vi "Preset_Edit.vi"() -> ()   [LabVIEW 2020, in "Gviewer.lvclass"]
doc: "Andre Koelewijn, 20 jan 2021\n\nEdit TAGs to display"
uses:
  Gviewer.lvclass
  controls/EditTagOneTag.ctl
  controls/Typedef_Gserver-Replies.ctl
  controls/Typedef_ServerActions.ctl
  DBAL/controls/DBAL_TAGprops.ctl
  DBAL/controls/DBAL_TAGpropEdit.ctl
  Common/controls/typedef_com_TagProp.ctl
  <vilib>/Utility/miscctls.llb/LVPointTypeDef.ctl
panel:
  in  "Exit_event":bool
  out "tag-info":string
  in  "TAGproperties":T1 {"TAGprop"."TagFunc" format="%08x"; "TAGprop"."RangeL" format="%.2f"; "TAGprop"."RangeH" format="%.2f"}
  in  "GViewer-Queue":refnum<queue>
  in  "SaveAs":bool
  in  "Save":bool
  in  "Cancel":bool
  in  "Selector":i32[](listbox)
  in  "Presets":T4[](array[typedef]) {"max" format="%#_6p"; "min" format="%#_6p"}
  # "Tag name"
  # "scale L"
  # "scale H"
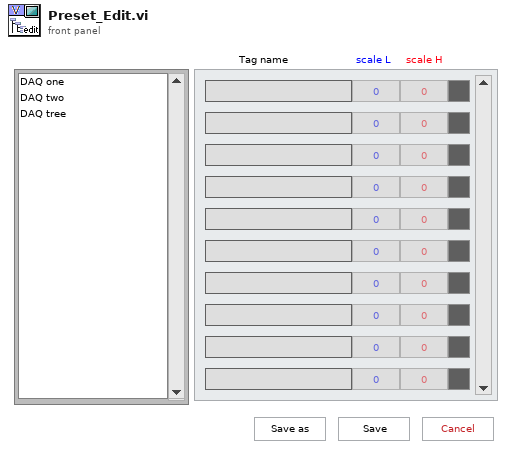
[diagram p1: front panel]
types:
  T1 = typedef "DBAL_TAGprops.ctl" = T2[]
  T2 = typedef "DBAL_TAGpropEdit.ctl" = cluster{"TAG":string, "Qtype":string, "TAGprop":T3}
  T3 = typedef "typedef_com_TagProp.ctl" = cluster{"Description":string, "EngUnits":string, "RangeH":dbl, "RangeL":dbl, "Resolution":i32, "Obsolete":bool, "ChangeDate":timestamp, "ChangeSource":string, "ChangeReason":string, "TagFunc":u32}
  T4 = typedef "EditTagOneTag.ctl" = cluster{"TAG":string, "min":dbl, "max":dbl, "Color":u32}
  T5 = typedef "LVPointTypeDef.ctl" = cluster{"Horizontal":i16, "Vertical":i16}
  T6 = typedef "Typedef_ServerActions.ctl" = enum16{"GraphUpdate", "SendAllTags", "SendIniPath", "SetGeneralOptions", "EditTagsOpen", "EditTagsClose", "NewTagSelection", "ExitGraph"}
  T7 = typedef "Typedef_Gserver-Replies.ctl" = cluster{"ServerActions":T6, "data":variant, "Source":string, "Time Stamp":timestamp}
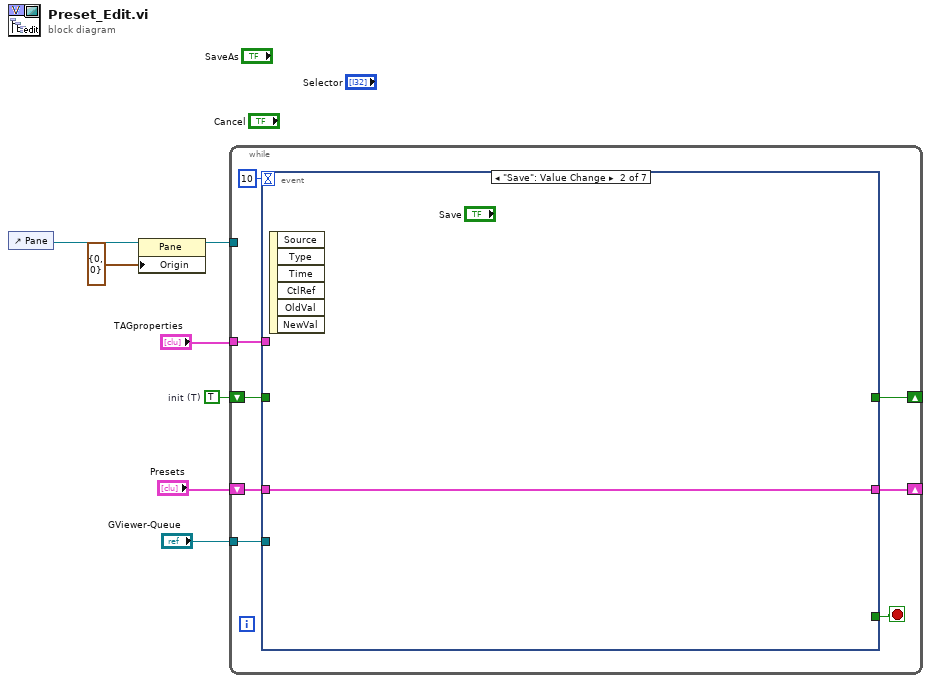
[diagram p0: block diagram]
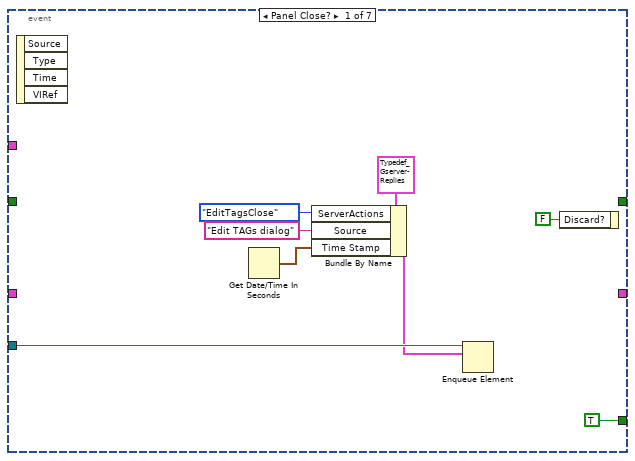
[diagram p2: hidden frame]
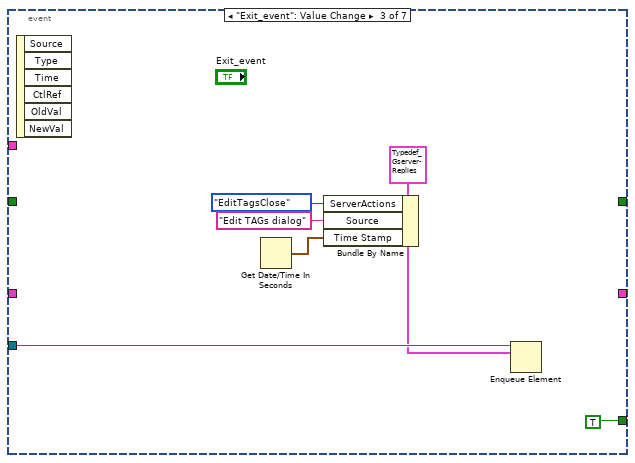
[diagram p3: hidden frame]
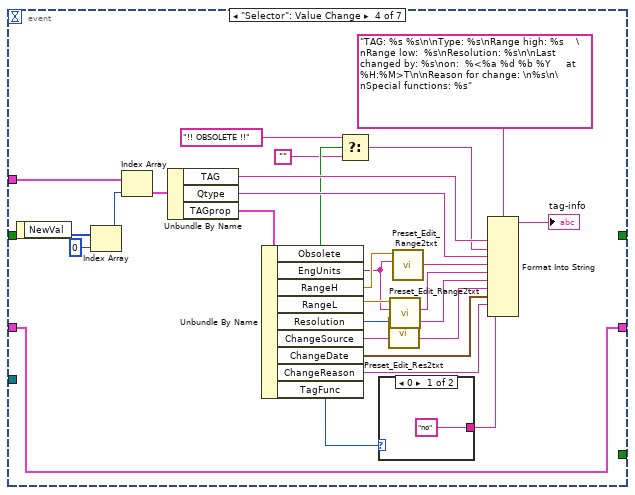
[diagram p4: hidden frame]
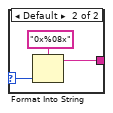
[diagram p5: hidden frame]
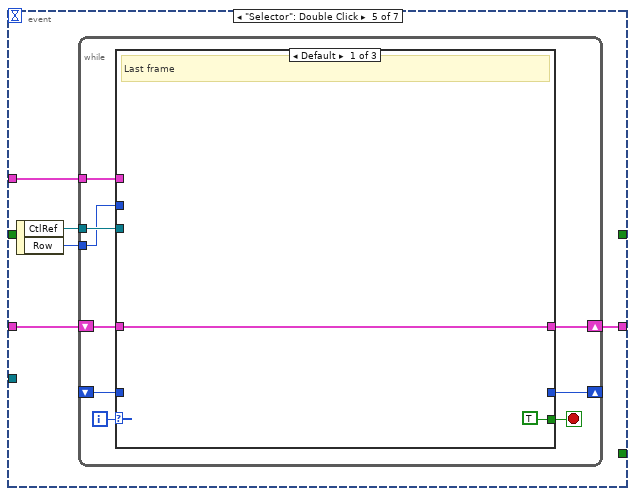
[diagram p6: hidden frame]
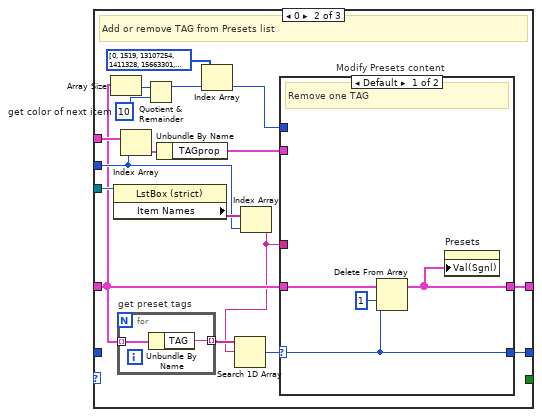
[diagram p7: hidden frame]
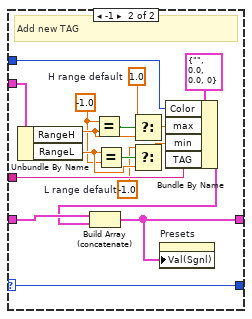
[diagram p8: hidden frame]
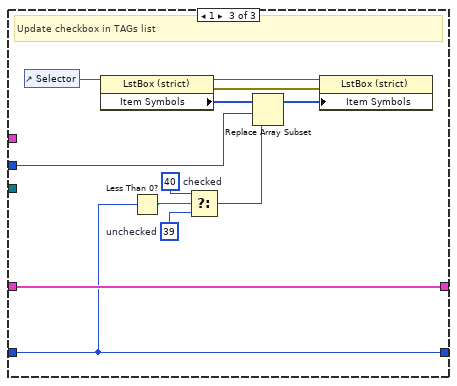
[diagram p9: hidden frame]
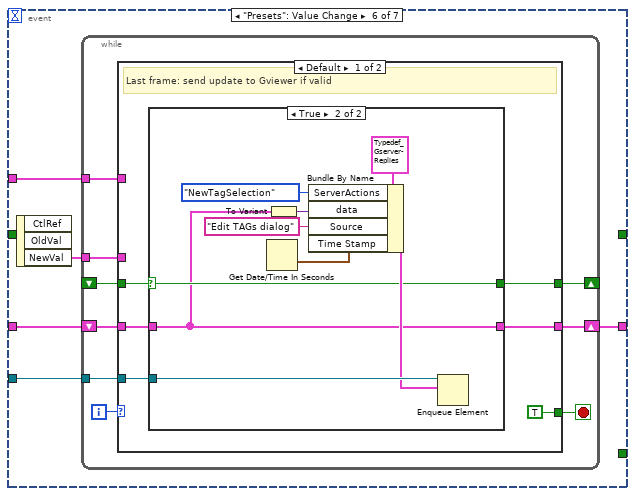
[diagram p10: hidden frame]
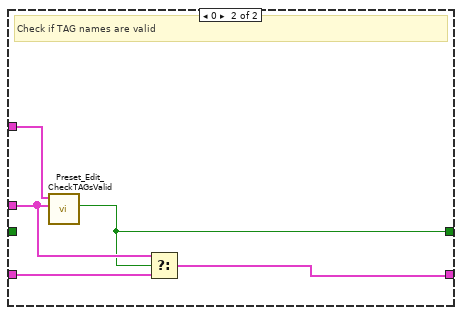
[diagram p12: hidden frame]
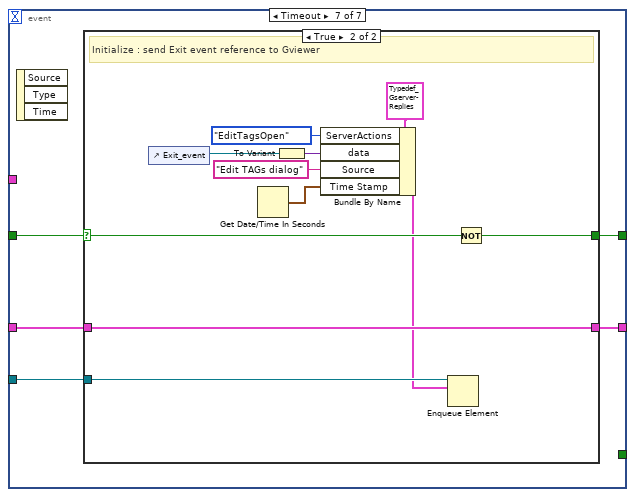
[diagram p13: hidden frame]
diagram:
  w1 = TRUE  # init (T)
  n1 = control-ref of="Pane"() -> (w6:refnum<vi>)
  n2 = property class="Pane"(reference=w6, "Origin"=T5 {"Horizontal"=0, "Vertical"=0}) -> (reference out=w5:refnum<vi>)  [unwired: 1 in, 1 out]
  n3 = while {
    tunnel: w5 -> [_]
    tunnel: "TAGproperties" -> [w13]
    tunnel: "GViewer-Queue" -> [w10]
    shift-right: [w11] -> _
    shift-left: "Presets" -> [w12]
    shift-right: [w8] -> _
    shift-left: w1 -> [w9]
    stop <- w15 stop-if-true
    n4 = event shown="[1] \"Save\": Value Change" {
      selector: _ -> [_ _ _ _ _ _ _]
      dyn-events: _ -> [_ _ _ _ _ _ _]
      timeout: 10 -> [_ _ _ _ _ _ _]
      tunnel: [TRUE _ TRUE _ _ _ _] -> w15
      tunnel: w13 -> [_ _ _ w57 w62 w130 _]
      tunnel: w12 -> [_ w24 _ w31 w64 w134 w169]
      tunnel: [_ w24 _ w31 w63 w133 w168] -> w11
      tunnel: w10 -> [w17 _ w29 _ _ w132 w166]
      tunnel: w9 -> [_ _ _ _ _ _ w170]
      tunnel: [_ _ _ _ _ _ w167] -> w8
      event Panel Close? {
        n5 = event-data() -> ()  [unwired: 1 in, 4 out]
        n6 = Get Date/Time In Seconds() -> (seconds since 1Jan1904=w21:timestamp)
        n7 = Bundle By Name(cluster=T7 {"ServerActions"=enum."GraphUpdate", "data"=variant, "Source"="", "Time Stamp"=timestamp(0 s since 1904-01-01)} ("element"), "ServerActions"=Typedef_ServerActions."EditTagsClose", "Source"="Edit TAGs dialog", "Time Stamp"=w21) -> (w16:T7)
        n8 = Enqueue Element(queue=w17, element=w16) -> ()  [unwired: 2 in, 3 out]
        n9 = event-data("Discard?"=FALSE) -> ()  [unwired: 1 in, 1 out]
      }
      event "Save": Value Change {
        n10 = event-data() -> ()  [unwired: 1 in, 6 out]
      }
      event "Exit_event": Value Change {
        w25 = T7 {"ServerActions"=enum."GraphUpdate", "data"=variant, "Source"="", "Time Stamp"=timestamp(0 s since 1904-01-01)} ("element")
        n11 = event-data() -> ()  [unwired: 1 in, 6 out]
        n12 = Get Date/Time In Seconds() -> (seconds since 1Jan1904=w26:timestamp)
        n13 = Bundle By Name(cluster=w25, "ServerActions"=Typedef_ServerActions."EditTagsClose", "Source"="Edit TAGs dialog", "Time Stamp"=w26) -> ()  [unwired: 1 out]
        n14 = Enqueue Element(queue=w29, element=w25) -> ()  [unwired: 2 in, 3 out]
      }
      event "Selector": Value Change {
        n15 = event-data() -> ("NewVal"=w56:i32[])  [unwired: 1 in]
        n16 = Index Array(array=w56, index=0) -> (element=w54:i32)
        n17 = Index Array(array=w57, index=w54) -> (element=w53:T2)
        n18 = Unbundle By Name(w53) -> ("TAG"=w44:string, "Qtype"=w50:string, "TAGprop"=w52:T3)
        n19 = Unbundle By Name(w52) -> ("Obsolete"=w43:bool, "EngUnits"=w37:string, "RangeH"=w39:dbl, "RangeL"=w38:dbl, "Resolution"=w35:i32, "ChangeSource"=w49:string, "ChangeDate"=w48:timestamp, "ChangeReason"=w47:string, "TagFunc"=w33:u32)
        n20 = Select(t="!! OBSOLETE !!" ("format string"), s=w43, f="") -> (s? t:f=w42:string)
        n21 = case shown="0" w33 {
          selector: w33 -> [_ w60]
          tunnel: ["no" w59] -> w32
          frame 0 {
          }
          frame Default {
            n22 = Format Into String(format string="0x%08x", w60) -> (resulting string=w59:string)  [unwired: 2 in, 1 out]
          }
        }
        n23 = call "Preset_Edit_Res2txt.vi"("Resolution"=w35) -> ("Resolution text"=w34:string)  [unwired: 10 in]
        n24 = call "Preset_Edit_Range2txt.vi"("Engineering units"=w37, "Range"=w38) -> ("RangeInfo"=w36:string)  [unwired: 9 in]
        n25 = call "Preset_Edit_Range2txt.vi"("Engineering units"=w37, "Range"=w39) -> ("RangeInfo"=w40:string)  [unwired: 9 in]
        n26 = Format Into String(format string="TAG: %s %s\n\nType: %s\nRange high: %s    \nRange low:  %s\nResolution: %s\n\nLast changed by: %s\non:  %<%a %d %b %Y     at  %H:%M>T\n\nReason for change: \n%s\n\nSpecial functions: %s", w44, w42, w50, w40, w36, w34, w49, w48, w47, w32) -> (resulting string=→"tag-info":string)  [unwired: 2 in, 1 out]
      }
      event "Selector": Double Click {
        n27 = event-data() -> ("CtlRef"=w66:refnum<vi>, "Row"=w65:i32)  [unwired: 1 in]
        n28 = while {
          tunnel: w66 -> [w71]
          tunnel: w65 -> [w70]
          shift-right: [w73] -> w63
          shift-left: w64 -> [w74]
          tunnel: w62 -> [w72]
          shift-right: [w69] -> _
          shift-left: _ -> [w68]
          i -> [w75]
          stop <- w67 stop-if-true
          n29 = case shown="Default" w75 {
            tunnel: w74 -> [w76 w83 w123]
            tunnel: [w76 w81 w123] -> w73
            tunnel: w72 -> [_ w87 _]
            tunnel: w71 -> [_ w88 _]
            tunnel: w70 -> [_ w86 w124]
            tunnel: [_ w78 w122] -> w69
            tunnel: w68 -> [_ _ w122]
            tunnel: [TRUE _ _] -> w67
            frame Default {
              # "Last frame"
            }
            frame 0 {
              w93 = 10  # get color of next item
              # "Add or remove TAG from Presets list"
              n30 = Array Size(array=w83) -> (size(s)=w94:i32)
              n31 = property class="LstBox (strict)"(reference=w88) -> ("Item Names"=w90:string[])  [unwired: 1 in, 2 out]
              n32 = for "get preset tags" {
                tunnel: w83 -> [w117] mode=indexing
                tunnel: [w116] -> w85 mode=indexing
                n33 = Unbundle By Name(w117) -> ("TAG"=w116:string)
              }
              n34 = Index Array(array=w87, index=w86) -> (element=w89:T2)
              n35 = Quotient & Remainder(x=w94, y=w93) -> (x-y*floor(x/y)=w91:i32)  [unwired: 1 out]
              n36 = Unbundle By Name(w89) -> ("TAGprop"=w80:T3)
              n37 = Index Array(array=u32[] [0, 1519, 13107254, 1411328, 15663301, 14444288, 40861, 6375227, 6783580, 10450432], index=w91) -> (element=w82:u32)
              n38 = Index Array(array=w90, index=w86) -> (element=w79:string)
              n39 = Search 1D Array(1D array=w85, element=w79) -> (index of element=w84:i32)  [unwired: 1 in]
              n40 = case "Modify Presets content" shown="Default" w84 {
                selector: w84 -> [w96 w100]
                tunnel: [w95 w99] -> w81
                tunnel: w83 -> [w97 w113]
                tunnel: w82 -> [_ w114]
                tunnel: w80 -> [_ w105]
                tunnel: w79 -> [_ w102]
                tunnel: [w96 w100] -> w78
                frame Default {
                  # "Remove one TAG"
                  n41 = Delete From Array(array=w97, length=1, index=w96) -> (array with subset deleted=w95:T4[])  [unwired: 1 out]
                  n42 = property on="Presets" class="Arr (strict)"("Val(Sgnl)"=w95) -> ()  [unwired: 2 in, 2 out]
                }
                frame -1 {
                  w101 = -1.0  # L range default
                  w108 = 1.0  # H range default
                  w107 = -1.0 ("x")
                  # "Add new TAG"
                  n43 = Unbundle By Name(w105) -> ("RangeH"=w112:dbl, "RangeL"=w111:dbl)
                  n44 = Equal?(x=w107, y=w112) -> (x = y?=w109:bool)
                  n45 = Equal?(x=w111, y=w107) -> (x = y?=w110:bool)
                  n46 = Select(t=w108, s=w109, f=w112) -> (s? t:f=w104:dbl)
                  n47 = Select(t=w101, s=w110, f=w111) -> (s? t:f=w103:dbl)
                  n48 = Bundle By Name(cluster=T4 {"TAG"="", "min"=0.0, "max"=0.0, "Color"=0} ("Selected-Tag"), "Color"=w114, "max"=w104, "min"=w103, "TAG"=w102) -> (w106:T4)
                  n49 = Build Array (concatenate)(w113, w106) -> (w99:T4[])
                  n50 = property on="Presets" class="Arr (strict)"("Val(Sgnl)"=w99) -> ()  [unwired: 2 in, 2 out]
                }
              }
            }
            frame 1 {
              w119 = 40  # checked
              w120 = 39  # unchecked
              # "Update checkbox in TAGs list"
              n51 = control-ref of="Selector"() -> (w129:refnum<vi>)
              n52 = property class="LstBox (strict)"(reference=w129) -> (reference out=w128:refnum<vi>, error out=w127:errorcluster, "Item Symbols"=w126:i32[])  [unwired: 1 in]
              n53 = Less Than 0?(x=w122) -> (x < 0?=w121:bool)
              n54 = Select(t=w119, s=w121, f=w120) -> (s? t:f=w118:i32)
              n55 = Replace Array Subset(array=w126, new element=w118, index=w124) -> (w125:i32[])
              n56 = property class="LstBox (strict)"(reference=w128, error in=w127, "Item Symbols"=w125) -> ()  [unwired: 2 out]
            }
          }
        }
      }
      event "Presets": Value Change {
        n57 = event-data() -> ("NewVal"=w131:T4[])  [unwired: 1 in, 2 out]
        n58 = while {
          shift-right: [w141] -> w133
          shift-left: w134 -> [w142]
          tunnel: w132 -> [w139]
          tunnel: w131 -> [w138]
          tunnel: w130 -> [w137]
          shift-right: [w136] -> _
          shift-left: _ -> [w135]
          i -> [w143]
          stop <- w140 stop-if-true
          n59 = case shown="Default" w143 {
            tunnel: w142 -> [w147 w164]
            tunnel: [w144 w162] -> w141
            tunnel: [TRUE _] -> w140
            tunnel: w139 -> [w148 _]
            tunnel: w138 -> [_ w163]
            tunnel: w137 -> [_ w165]
            tunnel: [w145 w161] -> w136
            tunnel: w135 -> [w146 _]
            frame Default {
              # "Last frame: send update to Gviewer if valid"
              n60 = case shown="True" w146 {
                selector: w146 -> [w151 w153]
                tunnel: w148 -> [_ w160]
                tunnel: w147 -> [w150 w152]
                tunnel: [w151 w153] -> w145
                tunnel: [w150 w152] -> w144
                frame False {
                }
                frame True {
                  n61 = Get Date/Time In Seconds() -> (seconds since 1Jan1904=w157:timestamp)
                  n62 = To Variant(anything=w152) -> (Variant=w154:variant)
                  n63 = Bundle By Name(cluster=T7 {"ServerActions"=enum."GraphUpdate", "data"=variant, "Source"="", "Time Stamp"=timestamp(0 s since 1904-01-01)} ("element"), "ServerActions"=Typedef_ServerActions."NewTagSelection", "data"=w154, "Source"="Edit TAGs dialog", "Time Stamp"=w157) -> (w158:T7)
                  n64 = Enqueue Element(queue=w160, element=w158) -> ()  [unwired: 2 in, 3 out]
                }
              }
            }
            frame 0 {
              # "Check if TAG names are valid"
              n65 = call "Preset_Edit_CheckTAGsValid.vi"("Presets-new"=w163, "TAGproperties"=w165) -> ("TAGs OK"=w161:bool)  [unwired: 8 in]
              n66 = Select(t=w163, s=w161, f=w164) -> (s? t:f=w162:T4[])
            }
          }
        }
      }
      event Timeout {
        n67 = event-data() -> ()  [unwired: 1 in, 3 out]
        n68 = case shown="True" w170 {
          selector: w170 -> [w171 w182]
          tunnel: w169 -> [w172 w183]
          tunnel: [w172 w183] -> w168
          tunnel: [w171 w181] -> w167
          tunnel: w166 -> [_ w180]
          frame False {
            # "normal idle operation"
          }
          frame True {
            # "Initialize : send Exit event reference to Gviewer"
            n69 = control-ref of="Exit_event"() -> (w177:refnum<vi>)
            n70 = Get Date/Time In Seconds() -> (seconds since 1Jan1904=w174:timestamp)
            n71 = To Variant(anything=w177) -> (Variant=w176:variant)
            n72 = Bundle By Name(cluster=T7 {"ServerActions"=enum."GraphUpdate", "data"=variant, "Source"="", "Time Stamp"=timestamp(0 s since 1904-01-01)} ("element"), "ServerActions"=Typedef_ServerActions."EditTagsOpen", "data"=w176, "Source"="Edit TAGs dialog", "Time Stamp"=w174) -> (w173:T7)
            n73 = Enqueue Element(queue=w180, element=w173) -> ()  [unwired: 2 in, 3 out]
            n74 = Not(x=w182) -> (.not. x?=w181:bool)
          }
        }
      }
    }
  }
